vi "Launch Manual Control Optimization.vi"(8 "error in":errorcluster, 10 "DeviceID":T1, 11 "SCADA in":refnum<class "EMS.lvclass">) -> (0 "error out":errorcluster, 3 "SCADA out":refnum<class "EMS.lvclass">)   [LabVIEW 2018, in "EMS Core.lvlib" / "EMS.lvclass"]
uses:
  EMS.lvclass
  C:/Users/Administrator/Desktop/LabVIEW EMS/EMS Generic Actor/EMS Generic/EMS Generic.lvclass
  C:/Program Files (x86)/National Instruments/LabVIEW 2018/vi.lib/ActorFramework/Actor/Actor.lvclass
  <vilib>/ORNL/CSEISMIC DDS/CSEISMIC DDS Base/Data Types/Controls/DeviceID.ctl
  Optimization/Manual Control Actor/Manual Control/Manual Control.lvclass
  C:/Users/Administrator/Desktop/LabVIEW EMS/Device Communication and Control Abstract Actor/Device Communication and Control Abstract/Device Communication and Control Abstract.lvclass
  EMS Messages/Pass Through Device Info Msg/Pass Through Device Info Msg.lvclass
  C:/Users/Administrator/Desktop/LabVIEW EMS/EMS Generic Actor/EMS Generic Messages/Return DER_Info Msg/Return DER_Info Msg.lvclass
  EMS Messages/Pass Through Device Measurement Msg/Pass Through Device Measurement Msg.lvclass
  C:/Users/Administrator/Desktop/LabVIEW EMS/EMS Generic Actor/EMS Generic Messages/Return DER_Measurement Msg/Return DER_Measurement Msg.lvclass
  EMS Messages/Pass Through Device Status Msg/Pass Through Device Status Msg.lvclass
  C:/Users/Administrator/Desktop/LabVIEW EMS/EMS Generic Actor/EMS Generic Messages/Return IED_Status Msg/Return IED_Status Msg.lvclass
  Optimization/Manual Control Actor/Manual Control/Manual Control.lvclass/Manual Control.ctl
  EMS Generic Actor/EMS Generic/EMS Generic.lvclass/EMS Generic.ctl
  EMS.lvclass/EMS.ctl
  <vilib>/ActorFramework/Actor/Actor.lvclass
  EMS Generic Actor/EMS Generic/EMS Generic.lvclass
  <vilib>/ORNL/CSEISMIC DDS/CSEISMIC DDS Base/CSEISMIC DDS.lvclass
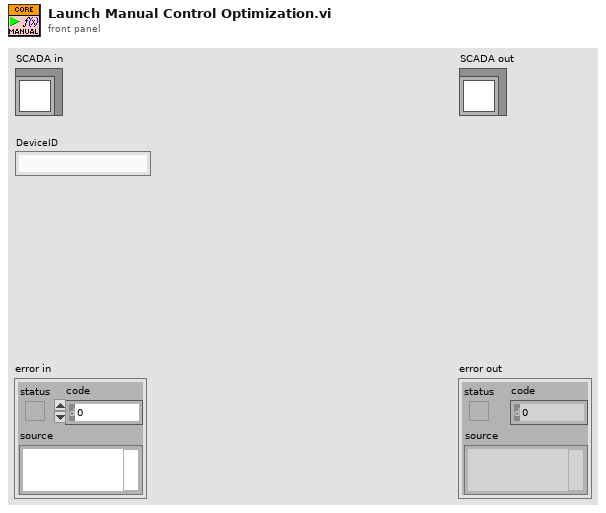
[diagram p1: front panel]
types:
  T1 = typedef "CSEISMIC DDS.lvlib/CSEISMIC DDS.lvclass/DeviceID.ctl" = string
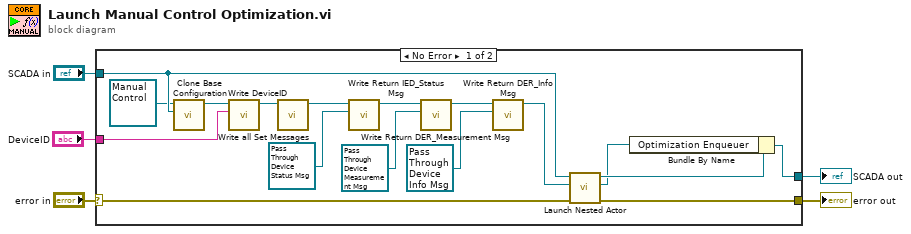
[diagram p0: block diagram]
diagram:
  n1 = case shown="No Error" "error in" {
    selector: "error in" -> [w18 w24]
    tunnel: [w21 w24] -> w4
    tunnel: [w20 w23] -> w2
    tunnel: "SCADA in" -> [w17 w23]
    tunnel: "DeviceID" -> [w15 _]
    frame No Error {
      n2 = call-dynamic "Clone Base Configuration.vi"("Source Object"=w17, "Target Object in"=refnum<class "Manual Control.lvclass"> refnum ("Manual Control Actor.lvlib:Manual Control.lvclass")) -> ("Target Object out"=w8:refnum<class "Manual Control.lvclass">)  [unwired: 9 in]
      n3 = call "Write DeviceID.vi"("DeviceID"=w15, "Manual Control in"=w8) -> ("Manual Control out"=w7:refnum<class "Manual Control.lvclass">)  [unwired: 9 in]
      n4 = call "Write all Set Messages.vi"("Device Communication and Control Abstract In"=w7) -> ("Device Communication and Control Abstract Out"=w6:refnum<class "Manual Control.lvclass">)  [unwired: 10 in]
      n5 = call "Write Return IED_Status Msg.vi"("Return IED_Status Msg"=refnum<class "Pass Through Device Status Msg.lvclass"> refnum ("SCADA Core.lvlib:Pass Through Device Status Msg.lvclass"), "EMS Generic in"=w6) -> ("EMS Generic out"=w14:refnum<class "Manual Control.lvclass">)  [unwired: 9 in]
      n6 = call "Write Return DER_Measurement Msg.vi"("Return DER_Measurement Msg"=refnum<class "Pass Through Device Measurement Msg.lvclass"> refnum ("SCADA Core.lvlib:Pass Through Device Measurement Msg.lvclass"), "EMS Generic in"=w14) -> ("EMS Generic out"=w13:refnum<class "Manual Control.lvclass">)  [unwired: 9 in]
      n7 = call "Write Return DER_Info Msg.vi"("Return DER_Info Msg"=refnum<class "Pass Through Device Info Msg.lvclass"> refnum ("SCADA Core.lvlib:Pass Through Device Info Msg.lvclass"), "EMS Generic in"=w13) -> ("EMS Generic out"=w12:refnum<class "Manual Control.lvclass">)  [unwired: 9 in]
      n8 = call <vilib>:"Launch Nested Actor.vi"("error in (no error)"=w18, "Nested Actor"=w12, "Caller Actor in"=w17) -> ("error out"=w21:errorcluster, "Nested Actor's Enqueuer"=w19:refnum<class "Message Enqueuer.lvclass">, "Caller Actor out"=w22:refnum<class "EMS.lvclass">)  [unwired: 6 in]
      n9 = Bundle By Name(cluster=w22, "Optimization Enqueuer"=w19) -> (w20:refnum<class "EMS.lvclass">)
    }
    frame Error {
    }
  }
  "error out" <- w4
  "SCADA out" <- w2
